vi "Power Accuracy Manage Strip Chart Display.vi"(7 "Clear?":bool, 10 "IM Power(s)":dbl[](array[numeric]), 11 "PIM Test Parameters":T1={"Stimulus"={"Power Start"=0, "Power Stop"=0, "Frequency Step Size"=enum."0.2", "TX 1 Frequency (MHz)"={"Min"=0.0, "Max"=0.0}, "TX 2 Frequency (MHz)"={"Min"=0.0, "Max"=0.0}, "RX Frequency (MHz)"={"Min"=0.0, "Max"=0.0}, "Pad Model Number"="", "Pad Serial Number"="", "Pad Values"=[]}, "Measurement"={"DUT Port"=enum."Port 1", "Direction"=0, "# Sweeps"=1}, "Display"={"Frequency"={"Min"=0.0, "Max"=0.0}, "Power"={"Min"=0, "Max"=0}, "Tolerance"={"Min"=0.0, "Max"=0.0}}, "Limit"={"Tolerance"=0.35}} {"Measurement"."Direction" items=["Reverse", "Forward", "Auxiliary"]}) -> (1 "Strip Total Span (seconds|samples)":dbl, 2 "Strip Window Span (seconds|samples)":dbl, 3 "PIM Traces":cluster{"x-values":dbl[], "y-values":dbl[]}[](array[cluster]), 5 "Point Plotted?":bool)   [LabVIEW 2011]
uses:
  SI.LIB/PIM.LIB/DISPLAY/Strip Chart Display Data.ctl
  SI.LIB/PIM.LIB/HW IO/MeasMode.ctl
  TypeDefs/Power Verification Test Parameters.ctl
  TypeDefs/Power Verification Display Parameters.ctl
  TypeDefs/Power Verification Measurement Parameters.ctl
  TypeDefs/Power Verification Stimulus Parameters.ctl
  SI.LIB/PIM.LIB/HW IO/DUTport.ctl
  TypeDefs/Power Verification Limit Parameters.ctl
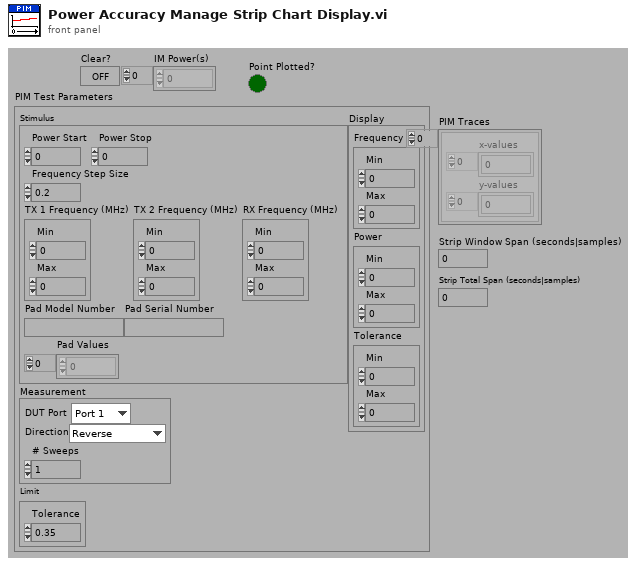
[diagram p1: front panel]
types:
  T1 = typedef "Power Verification Test Parameters.ctl" = cluster{"Stimulus":T2, "Measurement":T3, "Display":T6, "Limit":T7}
  T2 = typedef "Power Verification Stimulus Parameters.ctl" = cluster{"Power Start":i32, "Power Stop":i32, "Frequency Step Size":enum16{"0.2", "0.4", "1.0", "2.0", "4.0"}, "TX 1 Frequency (MHz)":cluster{"Min":dbl, "Max":dbl}, "TX 2 Frequency (MHz)":cluster{"Min":dbl, "Max":dbl}, "RX Frequency (MHz)":cluster{"Min":dbl, "Max":dbl}, "Pad Model Number":string, "Pad Serial Number":string, "Pad Values":dbl[]}
  T3 = typedef "Power Verification Measurement Parameters.ctl" = cluster{"DUT Port":T4, "Direction":T5, "# Sweeps":i32}
  T4 = typedef "DUTport.ctl" = enum16{"Port 1", "Port 2"}
  T5 = typedef "MeasMode.ctl" = u16
  T6 = typedef "Power Verification Display Parameters.ctl" = cluster{"Frequency":cluster{"Min":dbl, "Max":dbl}, "Power":cluster{"Min":i32, "Max":i32}, "Tolerance":cluster{"Min":dbl, "Max":dbl}}
  T7 = typedef "Power Verification Limit Parameters.ctl" = cluster{"Tolerance":dbl}
  T8 = typedef "Strip Chart Display Data.ctl" = cluster{"Reference Value":dbl, "Update Rate (s)":dbl, "Time Scale":dbl, "Hold":bool, "Clear":bool, "History Windows":i32, "HistoryView":bool}
  T9 = typedef "Power Verification Meas Units.ctl" = enum16{"Sample(s)", "Second(s)", "Sweep(s)"}
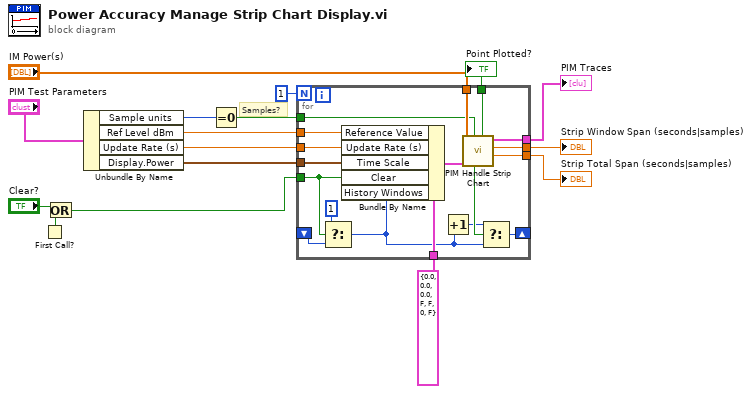
[diagram p0: block diagram]
diagram:
  # "Samples?"
  n1 = First Call?() -> (First Call?: T/F=w14:bool)
  n2 = Or(x="Clear?", y=w14) -> (x .or. y?=w12:bool)
  n3 = Unbundle By Name("PIM Test Parameters") -> ("Sample units"=w4:T9, "Ref Level dBm"=w5:dbl, "Update Rate (s)"=w2:dbl, "Display.Power"=w6:cluster{"Min":i32, "Max":i32})
  n4 = Equal To 0?(x=w4) -> (x = 0?=w3:bool)
  n5 = for {
    N: 1 -> [_]
    tunnel: T8 {"Reference Value"=0.0, "Update Rate (s)"=0.0, "Time Scale"=0.0, "Hold"=FALSE, "Clear"=FALSE, "History Windows"=0, "HistoryView"=FALSE} ("Strip Chart Display Data") -> [w34]
    tunnel: w6 -> [w33]
    tunnel: "IM Power(s)" -> [w32]
    tunnel: w12 -> [w28]
    tunnel: [w30] -> w11
    shift-right: [w23] -> _
    shift-left: _ -> [w27]
    tunnel: [w22] -> w10
    tunnel: [w21] -> w9
    tunnel: w5 -> [w20]
    tunnel: w3 -> [w19]
    tunnel: w2 -> [w18]
    tunnel: [w17] -> w1
    n6 = Select(t=1 ("Update Rate"), s=w28, f=w27) -> (s? t:f=w24:i32)
    n7 = Bundle By Name(cluster=w34, "Reference Value"=w20, "Update Rate (s)"=w18, "Time Scale"=w33, "Clear"=w28, "History Windows"=w24) -> (w31:T8)
    n8 = Increment(x=w24) -> (x+1=w25:i32)
    n9 = call "PIM Handle Strip Chart.vi"("Strip by sample? (F = seconds)"=w19, "Strip Chart Display Data"=w31, "Measured PIM (dBm/dBc)"=w32) -> ("Strip Total Span (seconds|samples)"=w21:dbl, "Strip Window Span (seconds|samples)"=w22:dbl, "PIM Traces"=w30:cluster{"x-values":dbl[], "y-values":dbl[]}[], "Point Plotted?"=w17:bool, "Increment History?"=w26:bool)  [unwired: 4 out]
    n10 = Select(t=w25, s=w26, f=w24) -> (s? t:f=w23:i32)
  }
  "PIM Traces" <- w11
  "Strip Window Span (seconds|samples)" <- w10
  "Strip Total Span (seconds|samples)" <- w9
  "Point Plotted?" <- w1
